vi "WildGruChil_V0.182.vi"() -> ()   [LabVIEW 2014]
uses:
  <vilib>/Utility/miscctls.llb/LVPointTypeDef.ctl
  <vilib>/Instr/_visa.llb/VISA Configure Serial Port (Instr).vi
  <vilib>/Utility/xml.llb/Read From XML File(string).vi
  <vilib>/Analysis/3filter.llb/IIR Filter (DBL).vi
  <vilib>/Utility/NIReport.llb/Append Report Text (str wrap).vi
  <vilib>/Utility/xml.llb/Write to XML File(string).vi
  <vilib>/Utility/NIReport.llb/NI_report.lvclass
  <vilib>/Analysis/NI_AALBase.lvlib
  <vilib>/gmath/NI_Gmath.lvlib
  <vilib>/Analysis/NI_AALPro.lvlib
panel:
  in  "min. Bytes":u32=15
  out "COM-Fehlerrate":string
  in  "nmax [1/min]":dbl=11000.0
  in  "nmin [1/min]":dbl=3000.0
  in  "Konfiguration:":bool
  in  "Speichern":bool
  in  "Drucken":bool
  out "Pmax":string="0,0 PS"
  in  "n vom Gas [1/min]":dbl=5000.0
  out "Ergebnis":string="0,0 PS bei 0 1/min   |   0,0 Nm bei 0 1/min   |   vmax: 2147483647 km/h\nDIN 70020 k =1,000 (20 °C, 50 %, 1013 mbar)\n20.11.2016 20:05 "
  in  "Fahrzeugdaten":string="Hier die Fahrzeugdaten eingeben"
  in  "Polynom":u8=15
  in  "Differenzenquotient":u8=12
  out "XY-Graph":cluster{dbl[], dbl[]}[](graph)
  in  "Rollenträgheit [kgm²]":dbl=0.402
  in  "[s]":dbl=5.0
  out "Untersetzung\nermittelt":bool
  out "Untersetzung":dbl format="%#.2f"
  in  "Reifenumfang [m]":dbl=1.222
  in  "Getriebe [1:]":dbl=5.343
  in  "Übersetzung ermitteln aus":bool=TRUE
  in  "Luftdruck [mbar]":dbl=1013.0
  in  "Luftfeuchtigkeit [%]":dbl=50.0
  in  "Lufttemperatur [°C]":dbl=20.0
  in  "Start [F1]":bool
  in  "Gl. Mittelwert":u8=35
  out "Füllstand Lesepuffer":u64(slide) scale=1.0..167.0
  out "Hinterrad\n[km/h]":dbl(knob) scale=0.0..150.0
  out "Welle\n[1/min]":cluster{dbl, dbl}(knob) scale=0.0..12000.0
  in  "Zündung [Imp/U]":u8=1
  in  "Rollenumfang [m]":dbl=0.613
  in  "Rolle [Inkr/U]":u16=200
  out "Lesepuffer":string="\n"
  in  "Serielle Schnittstelle":refnum<visa-resource-name>="COM6"
  in  "stop":bool
  out "Untersetzung-Graph":dbl(graph)=2.6802446808510636 caption="Untersetzung"
  # "1. n konstant halten\n2. START\n3. n weiter halten\n4. bei GO: Vollgas\n5. vom Gas gehen"
  # "Go"
  # "Zündsignal"
  # "Untersetzung:"
  # "Zündung\nRolle"
  # "Getriebe & Reifen"
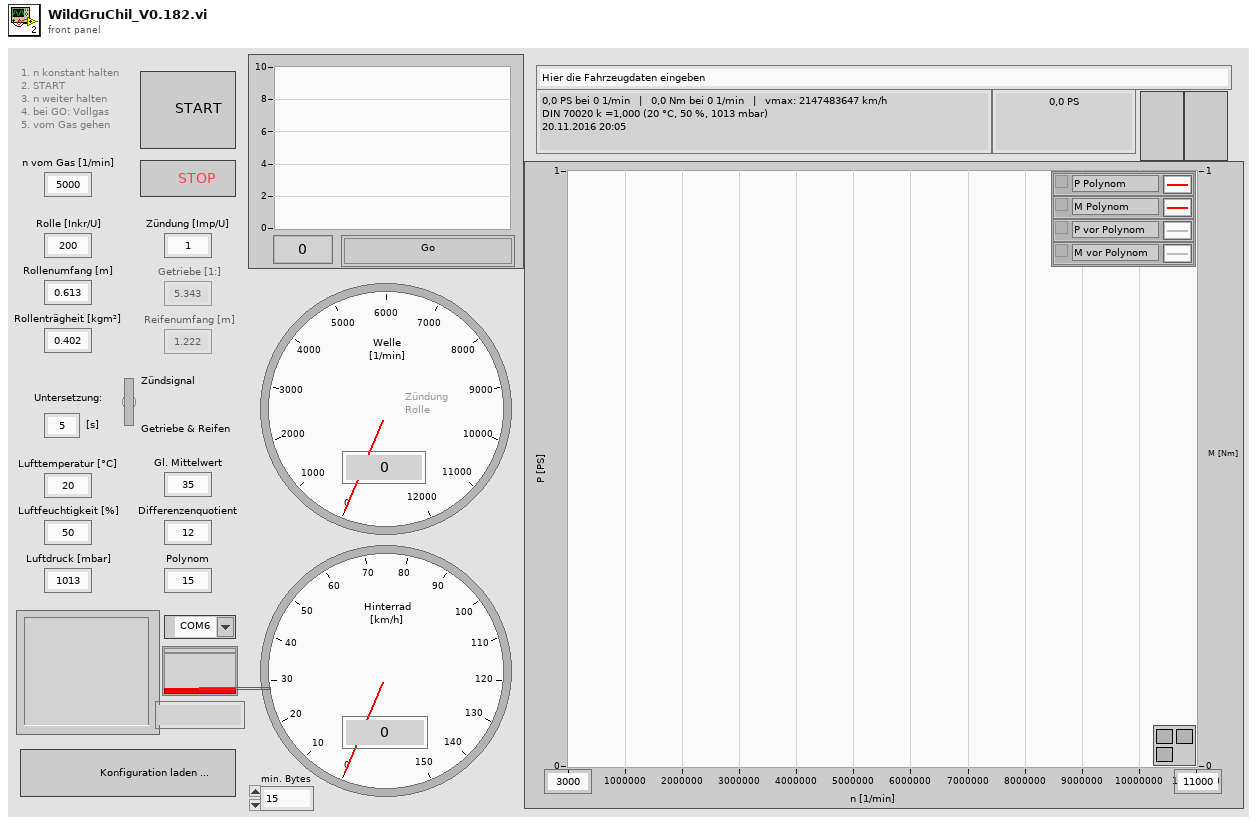
[diagram p1: front panel]
types:
  T1 = typedef "LVPointTypeDef.ctl" = cluster{"Horizontal":i16, "Vertical":i16}
  T2 = cluster{string, string, u16, dbl, dbl, u8, dbl, dbl, dbl, u8, u8, u8, dbl, dbl, dbl, dbl, dbl, dbl[], dbl[], dbl[], dbl[], bool, dbl, dbl, dbl, dbl, dbl[], i32[]}
  T3 = enum16{"Kleinste Quadrate", "Kleinestes absolutes Reiduum", "Biquadrat"}
  T4 = cluster{"Fahrzeugdaten":string, "date/time string":string, "Rolle [Inkr/U]":u16, "Rollenumfang [m]":dbl, "Rollenträgheit [kgm²]":dbl, "Zündung [Imp/U]":u8, "Getriebe [1:]":dbl, "Reifenumfang [m] ":dbl, "element":dbl, "Gl. Mittelwert":u8, "Differenzenquotient":u8, "Polynom":u8, "element":dbl, "element":dbl, "Lufttemperatur [°C]":dbl, "Luftfeuchtigkeit [%]":dbl, "Luftdruck [mbar]":dbl, dbl[], dbl[], "Best Polynomial Fit":dbl[], dbl[], "Übersetzung ermitteln aus":bool, "[s]":dbl, "nmin [1/min]":dbl, "nmax [1/min]":dbl, "n vom Gas [1/min]":dbl, dbl[], i32[]}
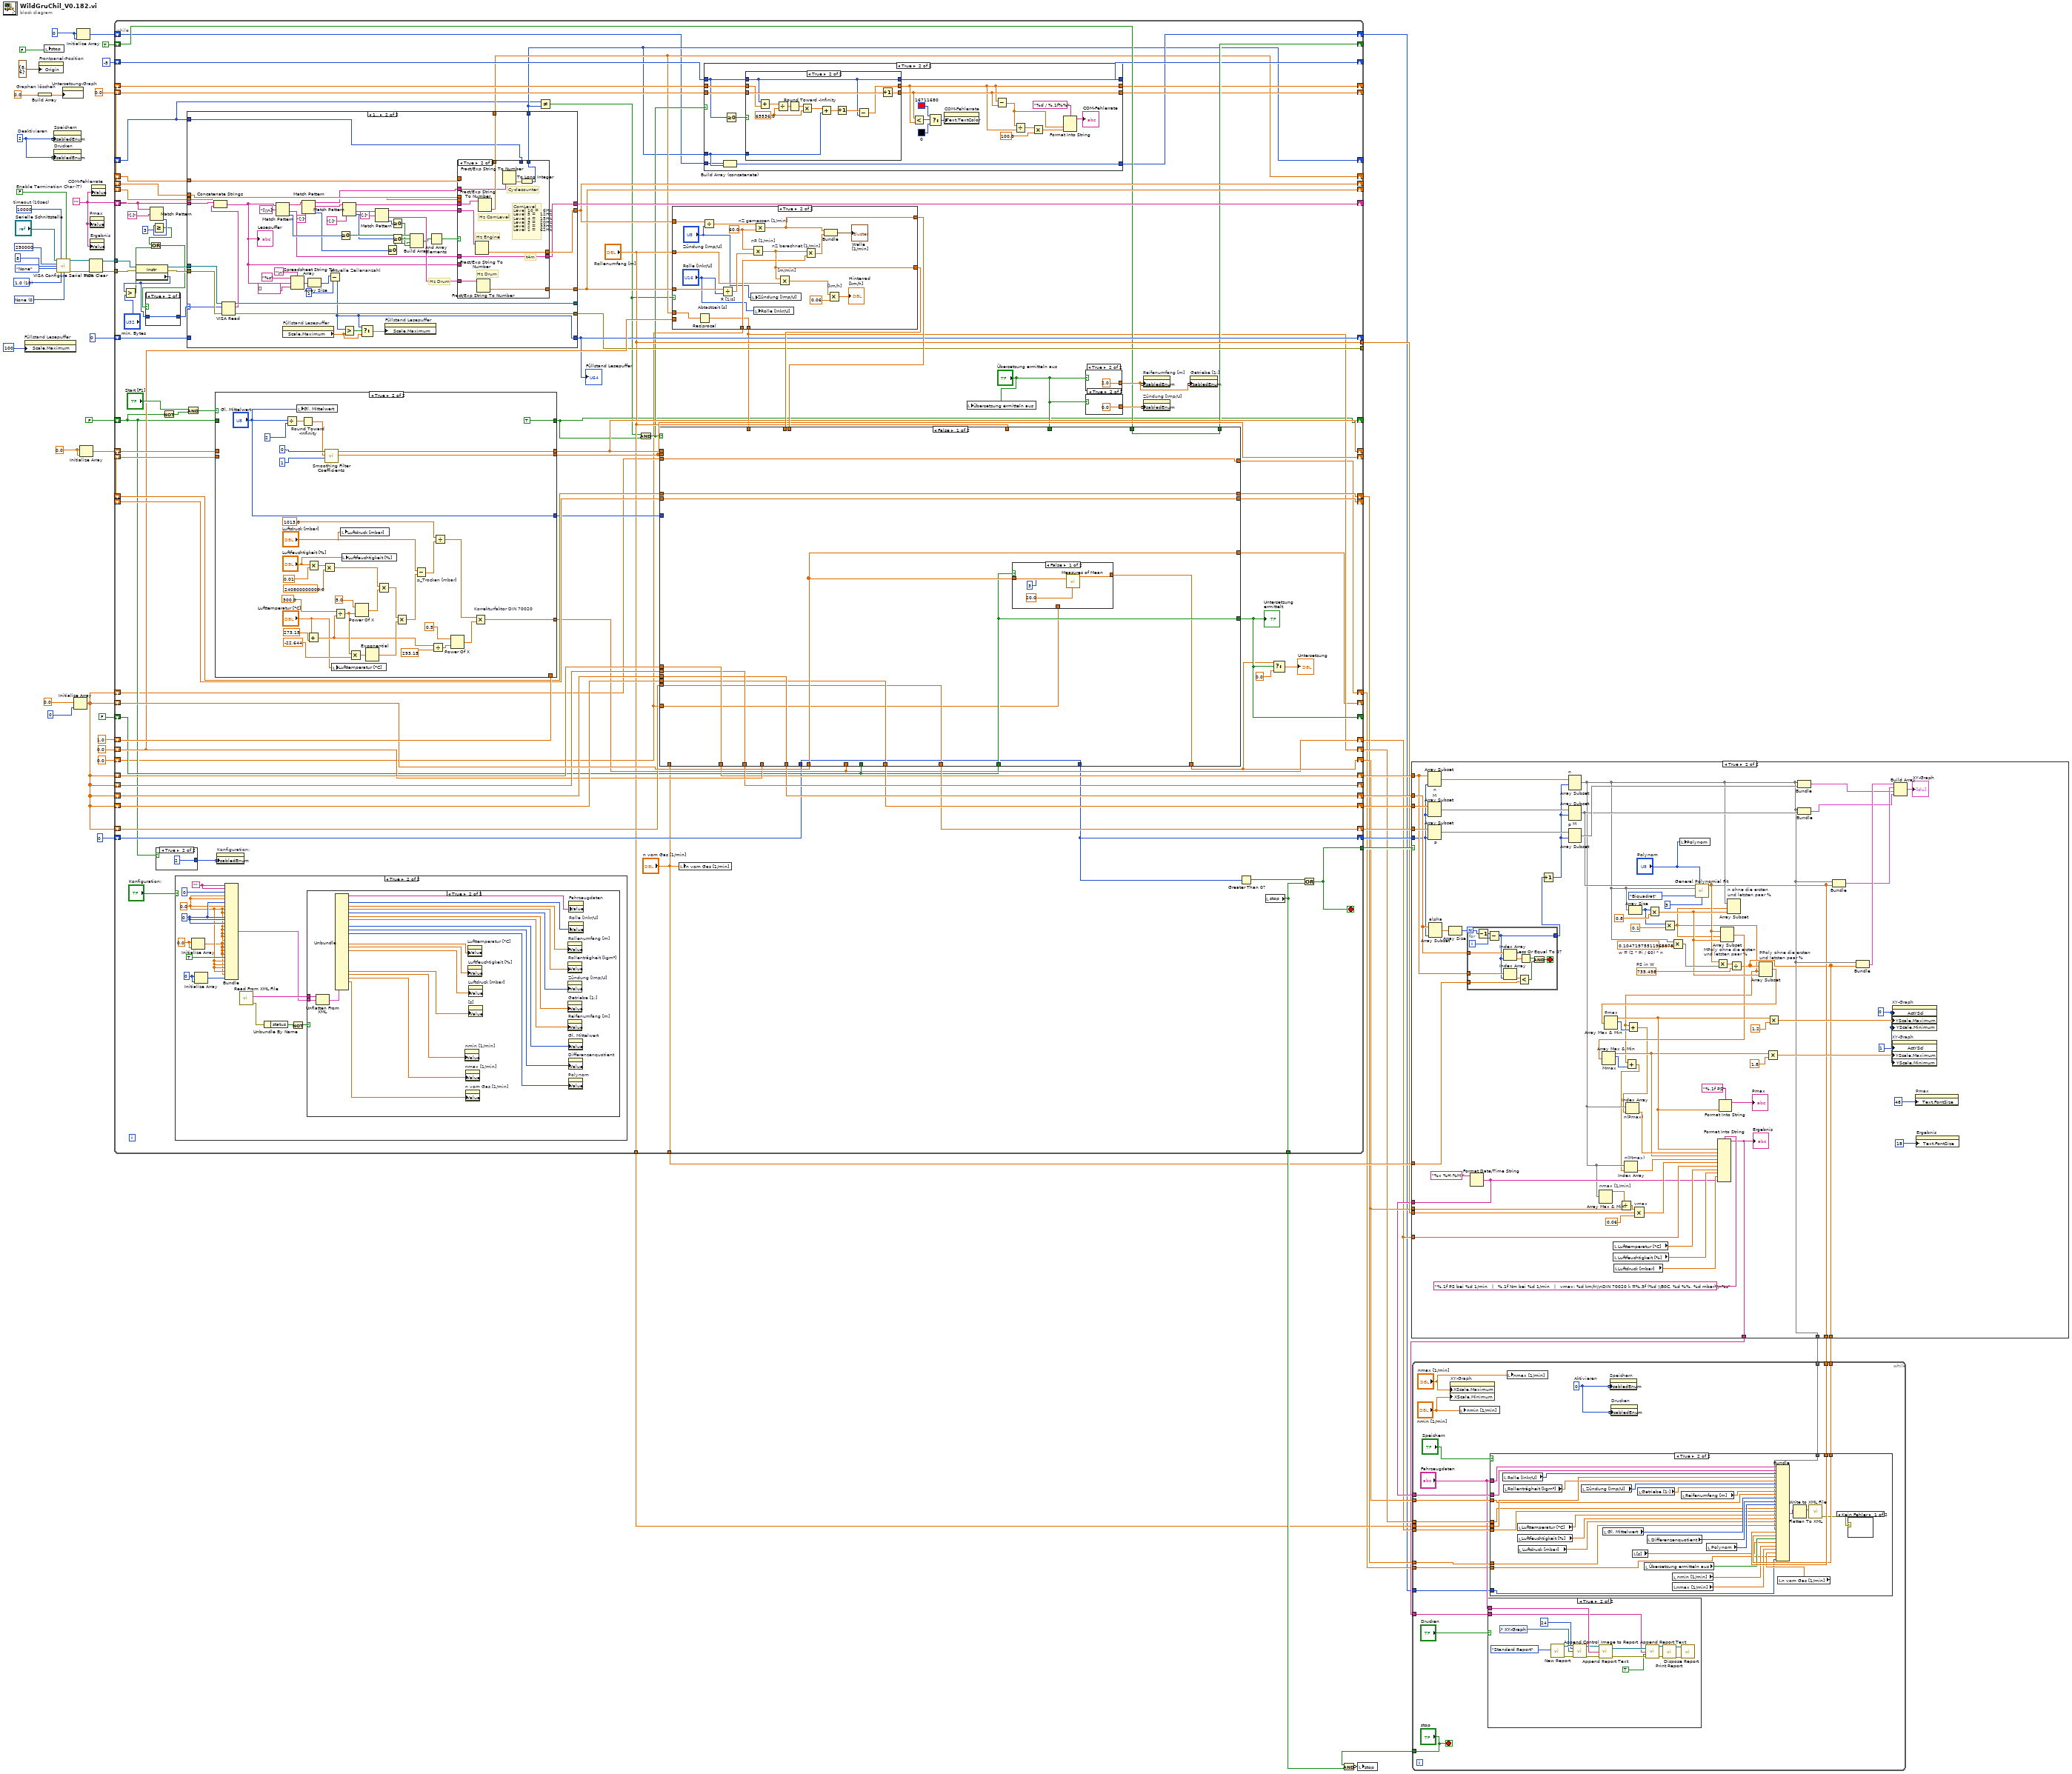
[diagram p0: block diagram]
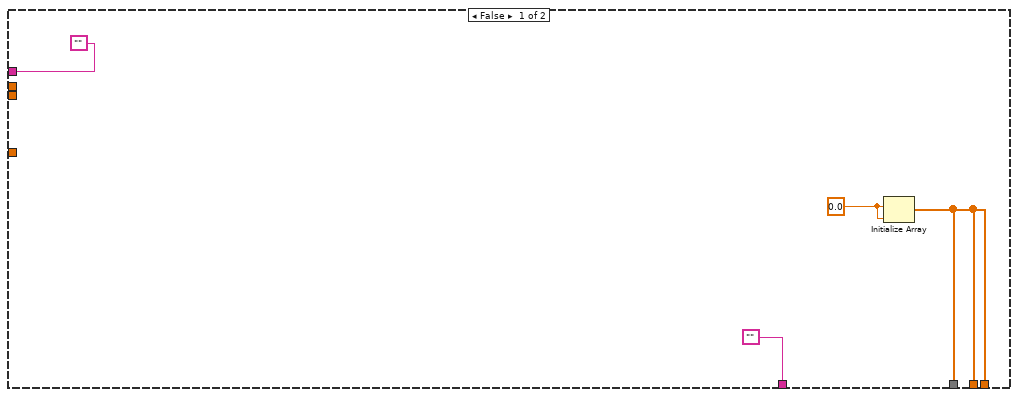
[diagram p5: hidden frame]
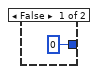
[diagram p6: hidden frame]
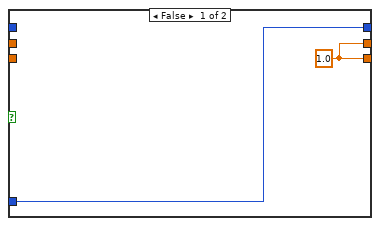
[diagram p8: hidden frame]
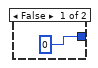
[diagram p11: hidden frame]
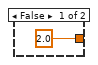
[diagram p12: hidden frame]
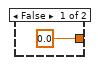
[diagram p13: hidden frame]
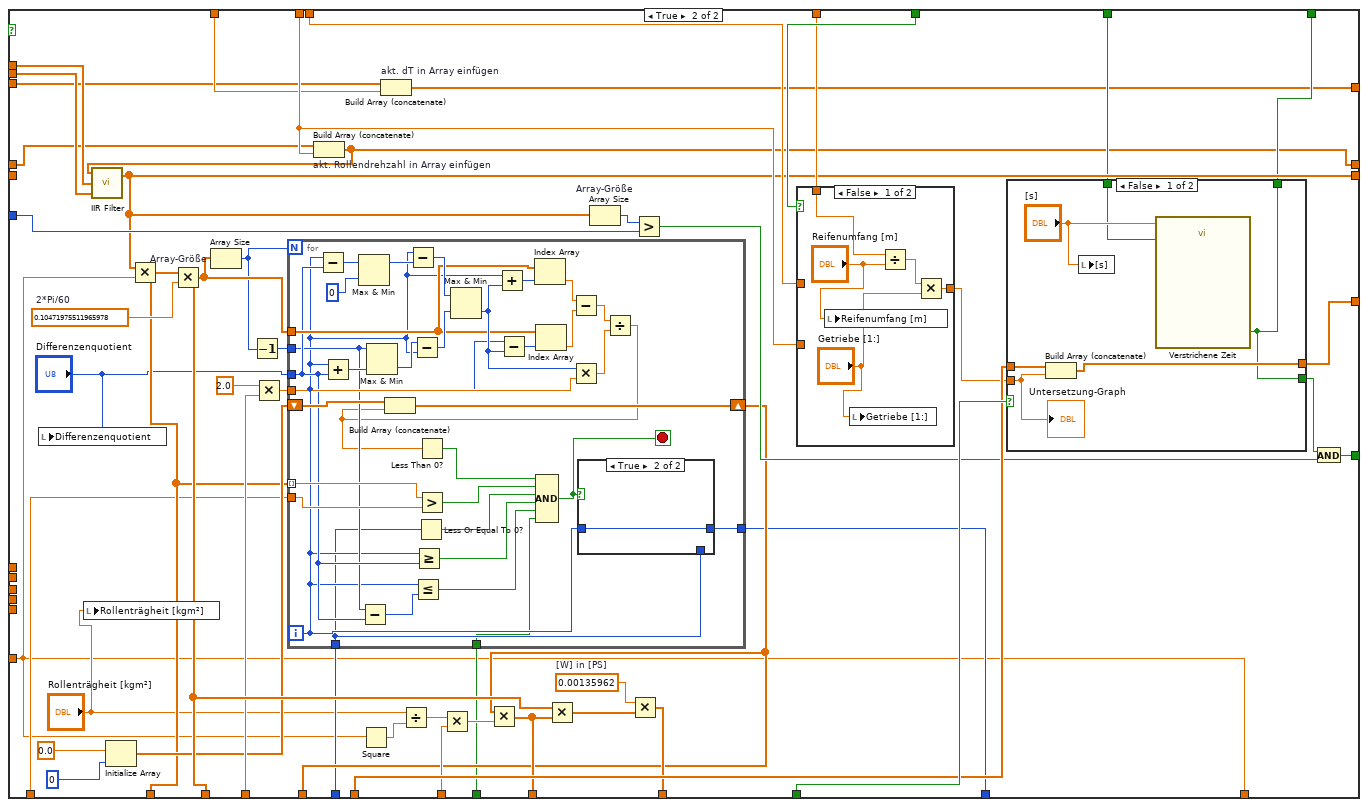
[diagram p15: hidden frame]
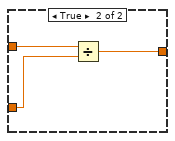
[diagram p18: hidden frame]
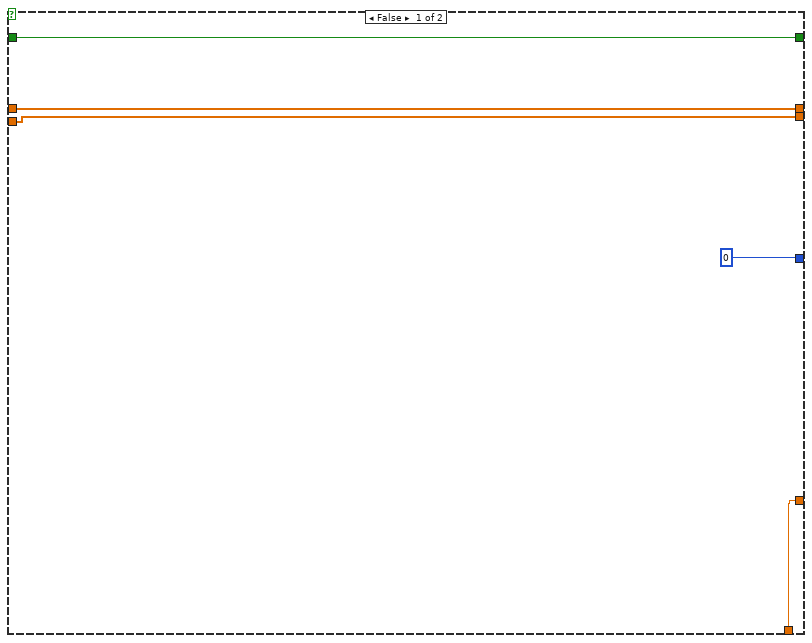
[diagram p19: hidden frame]
diagram:
  w6 = 0
  w2 = 0.0
  w11 = 2  # Deaktivieren
  w38 = 0.0
  w39 = 0.0  # Graphen löschen
  w54 = u16 0 items=["None", "XON/XOFF", "RTS/CTS", "XON/XOFF & RTS/CTS", "DTR/DSR", "XON/XOFF & DTR/DSR"] ("flow control (0:none)")
  w53 = u16 10 items=["1.0"=10, "1.5"=15, "2.0"=20] ("stop bits (10: 1 bit)")
  w3 = ""
  w58 = FALSE  # Enable Termination Char (T)
  w59 = u32 10000  # timeout (10sec)
  n1 = property on="Füllstand Lesepuffer" class="Schieber (strikt)"("Scale.Maximum"=100) -> ()  [unwired: 2 in, 2 out]
  n2 = Build Array(w39) -> (w36:dbl[])
  n3 = property on="Frontpanel-Position" class="Bereich"("Origin"=T1 {"Horizontal"=8, "Vertical"=6}) -> ()  [unwired: 2 in, 2 out]
  n4 = local write "stop"(FALSE) -> ()
  n5 = property on="Speichern" class="Bool."("DisabledEnum"=w11) -> ()  [unwired: 2 in, 2 out]
  n6 = property on="Drucken" class="Bool."("DisabledEnum"=w11) -> ()  [unwired: 2 in, 2 out]
  n7 = call-poly "VISA Configure Serial Port"("VISA resource name"="Serielle Schnittstelle", "timeout (10sec)"=w59, "Enable Termination\nChar (T)"=w58, "baud rate (9600)"=u32 250000 ("baudrate (250000)"), "data bits (8)"=u16 8, "parity (0:none)"=enum16{"None", "Odd", "Even", "Mark", "Space"}."None", "stop bits (10: 1 bit)"=w53, "flow control (0:none)"=w54) -> ("VISA resource name out"=w56:refnum<visa-resource-name>, "error out"=w57:errorcluster)  [unwired: 6 in]
  n8 = property on="Untersetzung-Graph" class="SVDiagr (strikt)"("History Data"=w36) -> ()  [unwired: 2 in, 2 out]
  n9 = Initialize Array(0.0 ("y"), 0) -> (w8:dbl[])
  n10 = Initialize Array(w6, w6) -> (w5:i32[])
  n11 = Initialize Array(w38, w38) -> (w37:dbl[])
  n12 = VISA Clear(VISA resource name=w56, error in (no error)=w57) -> (VISA resource name out=w51:refnum<visa-resource-name>, error out=w50:errorcluster)
  n13 = property on="Pmax" class="Str"("Value"=w3) -> ()  [unwired: 2 in, 2 out]
  n14 = property on="Ergebnis" class="Str"("Value"=w3) -> ()  [unwired: 2 in, 2 out]
  n15 = property on="COM-Fehlerrate" class="Str"("Value"=w3) -> ()  [unwired: 2 in, 2 out]
  n16 = while {
    tunnel: w51 -> [w149]
    tunnel: w50 -> [w148]
    shift-right: [w145] -> _
    shift-left: w3 -> [w65]
    shift-right: [w140] -> _
    shift-left: w2 -> [w144]
    shift-right: [w139] -> _
    shift-left: w2 -> [w143]
    shift-right: [w74] -> _
    shift-left: w2 -> [w142]
    shift-right: [w110] -> _
    shift-left: 0 -> [w141]
    shift-right: [w75] -> _
    shift-left: FALSE -> [w94]
    shift-right: [w105] -> w17
    shift-left: 1.0 ("element") -> [w133]
    shift-right: [w82] -> w22
    shift-left: 0.0 ("element") -> [w111]
    shift-right: [w126] -> w20
    shift-left: 0.0 ("element") -> [w77]
    shift-right: [w76] -> _
    shift-left: w8 -> [w130]
    shift-right: [w127] -> _
    shift-left: FALSE -> [w97]
    shift-right: [w125] -> _
    shift-left: w37 -> [w123]
    shift-right: [w124] -> _
    shift-left: w37 -> [w122]
    shift-right: [w121] -> w21
    shift-left: w37 -> [w119]
    shift-right: [w120] -> _
    shift-left: w37 -> [w118]
    shift-right: [w104] -> w29
    shift-left: w8 -> [w116]
    shift-right: [w109] -> _
    shift-left: w8 -> [w114]
    shift-right: [w108] -> w25
    shift-left: w8 -> [w115]
    shift-right: [w107] -> w28
    shift-left: w8 -> [w113]
    shift-right: [w106] -> w27
    shift-left: w8 -> [w112]
    tunnel: [w103] -> w35
    shift-right: [w98] -> w26
    shift-left: 0 -> [w100]
    tunnel: [w102] -> w31
    tunnel: [w101] -> _
    tunnel: ["n vom Gas [1/min]"] -> w24
    tunnel: ["Rollenumfang [m]"] -> w23
    tunnel: ["Rollenumfang [m]"] -> w15
    shift-right: [w89] -> _
    shift-left: TRUE -> [w90]
    shift-right: [w83] -> _
    shift-left: -5 -> [w88]
    shift-right: [w84] -> _
    shift-left: w2 -> [w87]
    shift-right: [w85] -> _
    shift-left: w2 -> [w86]
    shift-right: [w81] -> w7
    shift-left: w8 -> [w80]
    shift-right: [w73] -> _
    shift-left: _ -> [w72]
    shift-right: [w79] -> w4
    shift-left: w5 -> [w70]
    stop <- w103 stop-if-true
    n17 = property class="Instr"(reference=w149, error in=w148) -> (reference out=w146:refnum<visa-resource-name>, error out=w147:errorcluster, "Serial Settings:Number of Bytes at Serial Port"=w68:u32)
    n18 = Greater?(x=w68, y="min. Bytes") -> (0:w66:bool)
    n19 = Match Pattern(string=w65, regular expression="[;]") -> (offset past match=w63:i32)  [unwired: 1 in, 3 out]
    n20 = Greater Or Equal?(x=w63, y=3) -> (x >= y?=w62:bool)
    n21 = Or(x=w62, y=w66) -> (x .or. y?=w61:bool)
    n22 = case shown="True" w61 {
      tunnel: w68 -> [_ w151]
      tunnel: [u32 0 ("Bytes at Port") w151] -> w67
      frame False {
      }
      frame True {
      }
    }
    n23 = case shown="True" w94 {
      tunnel: [0 2] -> w93
      frame False {
      }
      frame True {
      }
    }
    n24 = Not(x=w94) -> (.not. x?=w138:bool)
    n25 = case shown="True" "Konfiguration:" {
      frame False {
      }
      frame True {
        w192 = 0
        w199 = u8 0
        w201 = 0.0
        w197 = 0.0
        w202 = ""
        n26 = Initialize Array(w201, w201) -> (w193:dbl[])
        n27 = Initialize Array(w192, w192) -> (w191:i32[])
        n28 = Bundle(w202, w202, u16 0, w197, w197, w199, w197, w197, w197, w199, w199, w199, w197, w197, w197, w197, w197, w193, w193, w193, w193, TRUE, w197, w197, w197, w197, w193, w191) -> (w203:T2)  [unwired: 1 in]
        n29 = call-poly <vilib>:"Read From XML File.vi"() -> ("error out"=w196:errorcluster, "XML Elements"=w204:string)  [unwired: 9 in, 1 out]
        n30 = Unbundle By Name(w196) -> ("status"=w194:bool)
        n31 = Not(x=w194) -> (.not. x?=w195:bool)
        n32 = case shown="True" w195 {
          tunnel: w204 -> [_ w224]
          tunnel: w203 -> [_ w223]
          frame False {
          }
          frame True {
            n33 = Unflatten From XML(xml string=w224, type=w223) -> (value=w222:T2)  [unwired: 1 in, 1 out]
            n34 = Unbundle(w222) -> (w221:string, w220:u16, w219:dbl, w218:dbl, w217:u8, w216:dbl, w215:dbl, w214:u8, w213:u8, w212:u8, w211:dbl, w210:dbl, w209:dbl, w208:dbl, w205:dbl, w206:dbl, w207:dbl)  [unwired: 11 out]
            n35 = property on="nmin [1/min]" class="DigWert (strikt)"("Value"=w205) -> ()  [unwired: 2 in, 2 out]
            n36 = property on="nmax [1/min]" class="DigWert (strikt)"("Value"=w206) -> ()  [unwired: 2 in, 2 out]
            n37 = property on="n vom Gas [1/min]" class="DigWert (strikt)"("Value"=w207) -> ()  [unwired: 2 in, 2 out]
            n38 = property on="Lufttemperatur [°C]" class="DigWert (strikt)"("Value"=w211) -> ()  [unwired: 2 in, 2 out]
            n39 = property on="Luftfeuchtigkeit [%]" class="DigWert (strikt)"("Value"=w210) -> ()  [unwired: 2 in, 2 out]
            n40 = property on="Luftdruck [mbar]" class="DigWert (strikt)"("Value"=w209) -> ()  [unwired: 2 in, 2 out]
            n41 = property on="[s]" class="DigWert (strikt)"("Value"=w208) -> ()  [unwired: 2 in, 2 out]
            n42 = property on="Rollenumfang [m]" class="DigWert (strikt)"("Value"=w219) -> ()  [unwired: 2 in, 2 out]
            n43 = property on="Rollenträgheit [kgm²]" class="DigWert (strikt)"("Value"=w218) -> ()  [unwired: 2 in, 2 out]
            n44 = property on="Zündung [Imp/U]" class="DigWert (strikt)"("Value"=w217) -> ()  [unwired: 2 in, 2 out]
            n45 = property on="Getriebe [1:]" class="DigWert (strikt)"("Value"=w216) -> ()  [unwired: 2 in, 2 out]
            n46 = property on="Reifenumfang [m]" class="DigWert (strikt)"("Value"=w215) -> ()  [unwired: 2 in, 2 out]
            n47 = property on="Gl. Mittelwert" class="DigWert (strikt)"("Value"=w214) -> ()  [unwired: 2 in, 2 out]
            n48 = property on="Differenzenquotient" class="DigWert (strikt)"("Value"=w213) -> ()  [unwired: 2 in, 2 out]
            n49 = property on="Polynom" class="DigWert (strikt)"("Value"=w212) -> ()  [unwired: 2 in, 2 out]
            n50 = property on="Fahrzeugdaten" class="Str"("Value"=w221) -> ()  [unwired: 2 in, 2 out]
            n51 = property on="Rolle [Inkr/U]" class="DigWert (strikt)"("Value"=w220) -> ()  [unwired: 2 in, 2 out]
          }
        }
      }
    }
    n52 = And(x="Start [F1]", y=w138) -> (x .and. y?=w137:bool)
    n53 = case shown="1.." w67 {
      selector: w67 -> [_ w463]
      tunnel: [w420 w457] -> w101
      tunnel: [w421 w458] -> _
      tunnel: w146 -> [w421 w465]
      tunnel: w147 -> [w420 w464]
      tunnel: [w417 w459] -> w139
      tunnel: [w418 w456] -> w140
      tunnel: w65 -> [w419 w454]
      tunnel: [w419 w452] -> w145
      tunnel: w144 -> [w418 w444]
      tunnel: w143 -> [w417 w443]
      tunnel: [w414 w442] -> w74
      tunnel: w142 -> [w414 w441]
      tunnel: w141 -> [w416 _]
      tunnel: [w416 w424] -> w110
      tunnel: [w415 w430] -> w73
      tunnel: w72 -> [w415 w429]
      frame 0, Default {
        # "No data in from serial port - Nothing to do."
      }
      frame 1.. {
        # "Hz Drum"
        n54 = VISA Read(VISA resource name=w465, byte count=w463, error in (no error)=w464) -> (VISA resource name out=w458:refnum<visa-resource-name>, read buffer=w455:string, error out=w457:errorcluster)  [unwired: 1 out]
        n55 = Concatenate Strings(w454, w455) -> (w426:string)
        "Lesepuffer" <- w426
        n56 = Match Pattern(string=w426, regular expression="[\\n]") -> (before substring=w433:string, after substring=w453:string, offset past match=w469:i32)  [unwired: 1 in, 1 out]
        n57 = property on="Füllstand Lesepuffer" class="Schieber (strikt)"() -> ("Scale.Maximum"=w423:dbl)  [unwired: 2 in, 2 out]
        n58 = Spreadsheet String To Array(delimiter (Tab)="\n" ("regular expression"), format string="%s" ("regular expression"), spreadsheet string=w426, array type (2D Dbl)=string[] [] ("Array 2")) -> (array=w435:string[])
        n59 = Match Pattern(string=w433, regular expression="[;]") -> (before substring=w431:string, after substring=w432:string, offset past match=w428:i32)  [unwired: 1 in, 1 out]
        n60 = Array Size(array=w435) -> (size(s)=w439:i32)
        n61 = Subtract "aktuelle Zeilenanzahl"(x=w439, y=1) -> (x-y=w424:i32)
        n62 = Greater Or Equal To 0?(x=w469) -> (x >= 0?=w451:bool)
        n63 = Match Pattern(string=w432, regular expression="[;]") -> (before substring=w462:string, after substring=w467:string, offset past match=w450:i32)  [unwired: 1 in, 1 out]
        n64 = Greater?(x=w424, y=w423) -> (0:w425:bool)
        n65 = Select(t=w424, s=w425, f=w423) -> (s? t:f=w422:dbl)
        n66 = Match Pattern(string=w467, regular expression="[;]") -> (before substring=w461:string, after substring=w460:string, offset past match=w448:i32)  [unwired: 1 in, 1 out]
        n67 = property on="Füllstand Lesepuffer" class="Schieber (strikt)"("Scale.Maximum"=w422) -> ()  [unwired: 2 in, 2 out]
        n68 = Greater Or Equal To 0?(x=w428) -> (x >= 0?=w427:bool)
        n69 = Greater Or Equal To 0?(x=w448) -> (x >= 0?=w447:bool)
        n70 = Greater Or Equal To 0?(x=w450) -> (x >= 0?=w449:bool)
        n71 = Build Array(w451, w449, w427, w447) -> (w446:bool[])
        n72 = And Array Elements(Boolean array=w446) -> (logical AND=w445:bool)
        n73 = case shown="True" w445 {
          tunnel: w462 -> [_ w480]
          tunnel: w461 -> [_ w485]
          tunnel: w460 -> [_ w484]
          tunnel: [w473 w483] -> w459
          tunnel: [w474 w482] -> w456
          tunnel: w453 -> [_ w481]
          tunnel: [w475 w481] -> w452
          tunnel: w426 -> [w475 _]
          tunnel: w444 -> [w474 _]
          tunnel: w443 -> [w473 _]
          tunnel: [w472 w479] -> w442
          tunnel: w441 -> [w472 _]
          tunnel: w431 -> [_ w478]
          tunnel: [w471 w476] -> w430
          tunnel: w429 -> [w471 _]
          frame False {
          }
          frame True {
            # "Cyclecounter"
            # "Hz ComLevel"
            # "ComLevel\nLevel 10 =   6Hz \nLevel 5 =   12Hz \nLevel 4 =   15Hz\nLevel 3 =   20Hz\nLevel 2 =   33Hz\nLevel 1 =   62Hz"
            # "Hz Drum"
            # "Hz Engine"
            # "t4m"
            n74 = Fract/Exp String To Number(string=w485) -> (number=w482:dbl)  [unwired: 3 in, 1 out]
            n75 = Fract/Exp String To Number(string=w484) -> (number=w483:dbl)  [unwired: 3 in, 1 out]
            n76 = Fract/Exp String To Number(string=w480) -> (number=w479:dbl)  [unwired: 3 in, 1 out]
            n77 = Fract/Exp String To Number(string=w478) -> (number=w477:dbl)  [unwired: 3 in, 1 out]
            n78 = To Long Integer(number=w477) -> (32bit integer=w476:i32)
          }
        }
      }
    }
    "Füllstand Lesepuffer" <- w110
    n79 = case shown="True" w137 {
      tunnel: [w357 TRUE] -> w75
      tunnel: w94 -> [w357 _]
      tunnel: [w356 w370] -> w105
      tunnel: w133 -> [w356 _]
      tunnel: [w355 w367] -> w125
      tunnel: [w354 w366] -> w124
      tunnel: w123 -> [w355 _]
      tunnel: w122 -> [w354 _]
      tunnel: [0 "Gl. Mittelwert"] -> w117
      frame False {
      }
      frame True {
        n80 = Divide(x="Gl. Mittelwert", y=2) -> (x/y=w365:dbl)
        n81 = local write "Gl. Mittelwert"("Gl. Mittelwert") -> ()
        n82 = Round Toward -Infinity(1:w365) -> (0:w364:dbl)
        n83 = Add(x="Lufttemperatur [°C]", y=273.15) -> (x+y=w376:dbl)
        n84 = Multiply(x="Luftfeuchtigkeit [%]", y=0.01) -> (x*y=w390:dbl)
        n85 = Multiply(x=w390, y=240800000000.0) -> (x*y=w361:dbl)
        n86 = call <vilib>:"Smoothing Filter Coefficients.vi"("shape"=1, "half-width"=w364, "type"=0) -> ("forward coefficients"=w366:dbl[], "reverse coefficients"=w367:dbl[])  [unwired: 6 in, 1 out]
        n87 = local write "Lufttemperatur [°C]"("Lufttemperatur [°C]") -> ()
        n88 = Divide ("M_Welle [Nm]")(x=300.0, y=w376) -> (x/y=w379:dbl)
        n89 = local write "Luftdruck [mbar]"("Luftdruck [mbar]") -> ()
        n90 = local write "Luftfeuchtigkeit [%]"("Luftfeuchtigkeit [%]") -> ()
        n91 = Multiply(x=w379, y=-22.644) -> (x*y=w385:dbl)
        n92 = Power Of X(1:w379, 2:5.0) -> (0:w377:dbl)
        n93 = Exponential(1:w385) -> (0:w383:dbl)
        n94 = Multiply(x=w361, y=w377) -> (x*y=w384:dbl)
        n95 = Multiply(x=w384, y=w383) -> (x*y=w382:dbl)
        n96 = Subtract "p_Trocken [mbar]"(x="Luftdruck [mbar]", y=w382) -> (x-y=w380:dbl)
        n97 = Divide ("M_Welle [Nm]")(x=w376, y=293.15) -> (x/y=w374:dbl)
        n98 = Divide ("M_Welle [Nm]")(x=1013.0, y=w380) -> (x/y=w372:dbl)
        n99 = Power Of X(1:w374, 2:0.5) -> (0:w371:dbl)
        n100 = Multiply "Korrekturfaktor DIN 70020"(x=w372, y=w371) -> (x*y=w370:dbl)
      }
    }
    n101 = property on="Konfiguration:" class="Bool."("DisabledEnum"=w93) -> ()  [unwired: 2 in, 2 out]
    n102 = Not Equal?(x=w72, y=w73) -> (x != y?=w71:bool)
    n103 = And(x=w71, y=w75) -> (x .and. y?=w78:bool)
    n104 = case "Case-Struktur" shown="True" w71 {
      tunnel: w140 -> [w395 w406]
      tunnel: w139 -> [w394 w405]
      tunnel: [w395 w404] -> w135
      tunnel: [w394 w403] -> w134
      tunnel: w74 -> [_ w397]
      tunnel: w111 -> [w393 _]
      tunnel: [w393 w396] -> w82
      tunnel: w77 -> [_ w402]
      tunnel: "Rollenumfang [m]" -> [_ w401]
      frame False {
      }
      frame True {
        w413 = 60.0 ("y")
        n105 = Reciprocal "Abtastzeit [s]"(x=w397) -> (1/x=w396:dbl)
        n106 = Divide(x=w406, y="Zündung [Imp/U]") -> (x/y=w409:dbl)
        n107 = Divide "R [1/s]"(x=w405, y="Rolle [Inkr/U]") -> (x/y=w412:dbl)
        n108 = local write "Zündung [Imp/U]"("Zündung [Imp/U]") -> ()
        n109 = Multiply "nR [1/min]"(x=w413, y=w412) -> (x*y=w403:dbl)
        n110 = Multiply "nZ gemessen [1/min]"(x=w409, y=w413) -> (x*y=w404:dbl)
        n111 = local write "Rolle [Inkr/U]"("Rolle [Inkr/U]") -> ()
        n112 = Multiply "[m/min]"(x=w403, y=w401) -> (x*y=w407:dbl)
        n113 = Multiply "nZ berechnet [1/min]"(x=w403, y=w402) -> (x*y=w411:dbl)
        n114 = Bundle(w404, w411) -> (→"Welle\n[1/min]":cluster{dbl, dbl})  [unwired: 1 in]
        n115 = Multiply "[km/h]"(x=w407, y=0.06) -> (x*y=→"Hinterrad\n[km/h]":dbl)
      }
    }
    n116 = case shown="False" w78 {
      tunnel: w135 -> [_ w291]
      tunnel: w134 -> [_ w290]
      tunnel: "Rollenumfang [m]" -> [_ w294]
      tunnel: [w242 w256] -> w126
      tunnel: w77 -> [w231 w256]
      tunnel: "Übersetzung ermitteln aus" -> [_ w299]
      tunnel: w97 -> [w243 w298]
      tunnel: w130 -> [w244 w297]
      tunnel: [w243 w268] -> w127
      tunnel: [w244 w296] -> w76
      tunnel: w125 -> [_ w293]
      tunnel: w124 -> [_ w292]
      tunnel: [w241 w253] -> w121
      tunnel: [w240 w267] -> w120
      tunnel: w119 -> [w241 w289]
      tunnel: w118 -> [w240 _]
      tunnel: w117 -> [_ w288]
      tunnel: [w239 w263] -> w104
      tunnel: w116 -> [w239 _]
      tunnel: [w238 w280] -> w109
      tunnel: w114 -> [w238 _]
      tunnel: w111 -> [_ w278]
      tunnel: [w237 w264] -> w108
      tunnel: w115 -> [w237 _]
      tunnel: [w236 w282] -> w107
      tunnel: w113 -> [w236 _]
      tunnel: [w235 w281] -> w106
      tunnel: w112 -> [w235 _]
      tunnel: w105 -> [_ w270]
      tunnel: w100 -> [w234 w262]
      tunnel: "n vom Gas [1/min]" -> [_ w261]
      tunnel: [w234 w260] -> w98
      tunnel: w97 -> [_ w259]
      tunnel: w90 -> [w233 w255]
      tunnel: [w233 w254] -> w89
      tunnel: w82 -> [_ w252]
      tunnel: [w232 w251] -> w81
      tunnel: w80 -> [w232 w250]
      frame False {
        n117 = case shown="False" w243 {
          tunnel: w244 -> [w248 _]
          tunnel: [w247 w249] -> w242
          tunnel: w231 -> [_ w249]
          frame False {
            n118 = call <vilib>:"Measures of Mean.vi"("percent (trim)"=20.0, "type"=3, "x array"=w248) -> ("mean value"=w247:dbl)  [unwired: 7 in, 1 out]
          }
          frame True {
          }
        }
      }
      frame True {
        w273 = 0.00135962  # [W] in [PS]
        w284 = 0.10471975511965978  # 2*Pi/60
        n119 = local write "Differenzenquotient"("Differenzenquotient") -> ()
        n120 = local write "Rollenträgheit [kgm²]"("Rollenträgheit [kgm²]") -> ()
        n121 = Initialize Array(0.0 ("y"), 0) -> (w274:dbl[])
        n122 = Multiply(x=2.0, y=w278) -> (x*y=w277:dbl)
        n123 = Build Array (concatenate) "akt. Rollendrehzahl in Array einfügen"(w289, w290) -> (w253:dbl[])
        n124 = call-poly <vilib>:"IIR Filter.vi"("Forward Coefficients"=w292, "Reverse Coefficients"=w293, "X"=w253) -> ("Filtered X"=w267:dbl[])  [unwired: 1 in, 1 out]
        n125 = Multiply(x=w267, y=w256) -> (x*y=w263:dbl[])
        n126 = Multiply(x=w263, y=w284) -> (x*y=w280:dbl[])
        n127 = Array Size "Array-Größe"(array=w280) -> (size(s)=w266:i32)
        n128 = Decrement(x=w266) -> (x-1=w265:i32)
        n129 = for {
          N: w266 -> [_]
          tunnel: "Differenzenquotient" -> [w311]
          tunnel: w280 -> [w319]
          tunnel: w265 -> [w310]
          tunnel: w277 -> [w320]
          shift-right: [w316] -> w264
          shift-left: w274 -> [w317]
          tunnel: w263 -> [w314] mode=indexing
          tunnel: w262 -> [w302]
          tunnel: w261 -> [w313]
          tunnel: [w303] -> w260
          tunnel: w259 -> [w300]
          i -> [w304]
          stop <- w301 stop-if-true
          n130 = Subtract(x=w304, y=w311) -> (x-y=w333:i32)
          n131 = Add(x=w304, y=w311) -> (x+y=w327:i32)
          n132 = Max & Min(x=w333, y=0) -> (max(x,y)=w331:i32)  [unwired: 1 out]
          n133 = Subtract(x=w310, y=w311) -> (x-y=w312:i32)
          n134 = Max & Min(x=w310, y=w327) -> (min(x,y)=w328:i32)  [unwired: 1 out]
          n135 = Subtract(x=w304, y=w331) -> (x-y=w330:i32)
          n136 = Subtract(x=w328, y=w304) -> (x-y=w329:i32)
          n137 = Less Or Equal?(x=w304, y=w312) -> (x <= y?=w308:bool)
          n138 = Greater Or Equal?(x=w304, y=w311) -> (x >= y?=w307:bool)
          n139 = Less Or Equal To 0?(x=w302) -> (x <= 0?=w305:bool)
          n140 = Greater?(x=w314, y=w313) -> (0:w315:bool)
          n141 = Max & Min(x=w330, y=w329) -> (min(x,y)=w321:i32)  [unwired: 1 out]
          n142 = Add(x=w304, y=w321) -> (x+y=w326:i32)
          n143 = Subtract(x=w304, y=w321) -> (x-y=w325:i32)
          n144 = Index Array(array=w319, index=w326) -> (element=w323:dbl)
          n145 = Index Array(array=w319, index=w325) -> (element=w324:dbl)
          n146 = Subtract(x=w323, y=w324) -> (x-y=w322:dbl)
          n147 = Multiply(x=w321, y=w320) -> (x*y=w318:dbl)
          n148 = Divide(x=w322, y=w318) -> (x/y=w309:dbl)
          n149 = Build Array (concatenate)(w317, w309) -> (w316:dbl[])
          n150 = Less Than 0?(x=w309) -> (x < 0?=w306:bool)
          n151 = Compound Arithmetic op=AND(w306, w315, w305, w307, w308, w300) -> (w301:bool)
          n152 = case shown="True" w301 {
            tunnel: w304 -> [_ w335]
            tunnel: [w334 w335] -> w303
            tunnel: w302 -> [w334 _]
            frame False {
            }
            frame True {
            }
          }
        }
        n153 = Square(x=w256) -> (x^2=w283:dbl)
        n154 = Build Array (concatenate) "akt. dT in Array einfügen"(w250, w252) -> (w251:dbl[])
        n155 = Divide(x="Rollenträgheit [kgm²]", y=w283) -> (x/y=w271:dbl)
        n156 = Multiply(x=w271, y=w270) -> (x*y=w269:dbl)
        n157 = Multiply(x=w264, y=w269) -> (x*y=w282:dbl[])
        n158 = Multiply(x=w280, y=w282) -> (x*y=w272:dbl[])
        n159 = Array Size "Array-Größe"(array=w267) -> (size(s)=w285:i32)
        n160 = Multiply(x=w273, y=w272) -> (x*y=w281:dbl[])
        n161 = Greater?(x=w285, y=w288) -> (0:w286:bool)
        n162 = case shown="False" w299 {
          tunnel: w291 -> [_ w352]
          tunnel: w290 -> [_ w351]
          tunnel: [w348 w350] -> w295
          tunnel: w294 -> [w349 _]
          frame False {
            n163 = local write "Reifenumfang [m]"("Reifenumfang [m]") -> ()
            n164 = local write "Getriebe [1:]"("Getriebe [1:]") -> ()
            n165 = Divide(x=w349, y="Reifenumfang [m]") -> (x/y=w347:dbl)
            n166 = Multiply(x=w347, y="Getriebe [1:]") -> (x*y=w348:dbl)
          }
          frame True {
            n167 = Divide(x=w352, y=w351) -> (x/y=w350:dbl)
          }
        }
        n168 = case shown="False" w298 {
          selector: w298 -> [_ w344]
          tunnel: w295 -> [w339 _]
          tunnel: w297 -> [w341 w343]
          tunnel: [w336 w344] -> w287
          tunnel: [w340 w343] -> w296
          tunnel: w255 -> [w337 w342]
          tunnel: [w336 w342] -> w254
          frame False {
            n169 = Build Array (concatenate)(w341, w339) -> (w340:dbl[])
            n170 = local write "[s]"("[s]") -> ()
            n171 = call "Verstrichene Zeit"("Time Target (s)"="[s]", "Reset"=w337) -> ("Time has Elapsed"=w336:bool)  [unwired: 10 in, 7 out]
            "Untersetzung-Graph" <- w339
          }
          frame True {
          }
        }
        n172 = And(x=w287, y=w286) -> (x .and. y?=w268:bool)
      }
    }
    "Untersetzung\nermittelt" <- w127
    n173 = local write "n vom Gas [1/min]"("n vom Gas [1/min]") -> ()
    n174 = case shown="True" w78 {
      tunnel: w88 -> [w155 w162]
      tunnel: [w155 w175] -> w83
      tunnel: w87 -> [w154 w174]
      tunnel: [w154 w158] -> w84
      tunnel: w86 -> [w153 w173]
      tunnel: [w153 w159] -> w85
      tunnel: w73 -> [_ w157]
      tunnel: w70 -> [w152 w156]
      tunnel: [w152 w161] -> w79
      frame False {
      }
      frame True {
        n175 = Build Array (concatenate)(w156, w157) -> (w161:i32[])
        n176 = Greater Or Equal To 0?(x=w162) -> (x >= 0?=w163:bool)
        n177 = case shown="True" w163 {
          tunnel: [w176 w187] -> w158
          tunnel: [w176 w188] -> w159
          tunnel: [w177 w179] -> w175
          tunnel: w174 -> [_ w181]
          tunnel: w173 -> [_ w189]
          tunnel: w157 -> [w177 w178]
          tunnel: w162 -> [_ w179]
          frame False {
            w176 = 1.0
          }
          frame True {
            w185 = 65536.0
            n178 = Add(x=w179, y=w181) -> (x+y=w180:dbl)
            n179 = Divide(x=w180, y=w185) -> (x/y=w190:dbl)
            n180 = Round Toward -Infinity(1:w190) -> (0:w186:dbl)
            n181 = Multiply(x=w186, y=w185) -> (x*y=w184:dbl)
            n182 = Add(x=w184, y=w178) -> (x+y=w183:dbl)
            n183 = Increment(x=w183) -> (x+1=w182:dbl)
            n184 = Subtract(x=w182, y=w179) -> (x-y=w187:dbl)
            n185 = Increment(x=w189) -> (x+1=w188:dbl)
          }
        }
        n186 = Less?(x=w159, y=w158) -> (x < y?=w171:bool)
        n187 = Select(t=u32 16711680, s=w171, f=u32 0) -> (s? t:f=w167:u32)
        n188 = property on="COM-Fehlerrate" class="Str"("Text.TextColor"=w167) -> ()  [unwired: 2 in, 2 out]
        n189 = Subtract(x=w158, y=w159) -> (x-y=w160:dbl)
        n190 = Divide(x=w160, y=w158) -> (x/y=w166:dbl)
        n191 = Multiply(x=w166, y=100.0) -> (x*y=w164:dbl)
        n192 = Format Into String(format string="%d / %.1f%%" ("Format-String"), w160, w164) -> (resulting string=→"COM-Fehlerrate":string)  [unwired: 2 in, 1 out]
      }
    }
    n193 = local write "Übersetzung ermitteln aus"("Übersetzung ermitteln aus") -> ()
    n194 = case shown="True" "Übersetzung ermitteln aus" {
      tunnel: [0.0 ("y") 2.0 ("y")] -> w131
      frame False {
      }
      frame True {
      }
    }
    n195 = case shown="True" "Übersetzung ermitteln aus" {
      tunnel: [2.0 ("y") 0.0 ("y")] -> w132
      frame False {
      }
      frame True {
      }
    }
    n196 = property on="Reifenumfang [m]" class="DigWert (strikt)"("DisabledEnum"=w131) -> ()  [unwired: 2 in, 2 out]
    n197 = property on="Zündung [Imp/U]" class="DigWert (strikt)"("DisabledEnum"=w132) -> ()  [unwired: 2 in, 2 out]
    n198 = property on="Getriebe [1:]" class="DigWert (strikt)"("DisabledEnum"=w131) -> ()  [unwired: 2 in, 2 out]
    n199 = Greater Than 0?(x=w98) -> (x > 0?=w99:bool)
    n200 = local read "stop"() -> (w102:bool)
    n201 = Select(t=w126, s=w127, f=0.0) -> (s? t:f=→"Untersetzung":dbl)
    n202 = Or(x=w99, y=w102) -> (x .or. y?=w103:bool)
  }
  n203 = case shown="True" w35 {
    tunnel: w29 -> [_ w547]
    tunnel: w28 -> [_ w552]
    tunnel: w27 -> [_ w551]
    tunnel: w26 -> [_ w523]
    tunnel: w25 -> [_ w548]
    tunnel: w24 -> [_ w546]
    tunnel: w23 -> [_ w540]
    tunnel: w17 -> [_ w526]
    tunnel: ["" w525] -> w18
    tunnel: w20 -> [_ w524]
    tunnel: ["" w522] -> w16
    tunnel: [w486 w499] -> w14
    tunnel: [w486 w498] -> w13
    tunnel: [w486 w497] -> w12
    frame False {
      w487 = 0.0
      n204 = Initialize Array(w487, w487) -> (w486:dbl[])
    }
    frame True {
      w511 = 735.498  # PS in W
      w517 = 0.10471975511965978  # w = (2 * Pi / 60) * n
      w521 = 0
      n205 = Array Subset "n"(array=w547, length=w523) -> (w545:dbl[])  [unwired: 1 in]
      n206 = Array Subset "M"(array=w552, length=w523) -> (w544:dbl[])  [unwired: 1 in]
      n207 = Array Subset "P"(array=w551, length=w523) -> (w543:dbl[])  [unwired: 1 in]
      n208 = Array Subset "alpha"(array=w548, length=w523) -> (w549:dbl[])  [unwired: 1 in]
      n209 = Array Size(array=w549) -> (size(s)=w550:i32)
      n210 = for {
        N: w550 -> [w570]
        tunnel: w548 -> [w567]
        tunnel: w547 -> [w564]
        tunnel: w546 -> [w561]
        tunnel: [w559] -> w519
        i -> [w565]
        stop <- w560 stop-if-true
        n211 = Decrement(x=w570) -> (x-1=w569:i32)
        n212 = Subtract(x=w569, y=w565) -> (x-y=w559:i32)
        n213 = Index Array(array=w567, index=w559) -> (element=w568:dbl)
        n214 = Index Array(array=w564, index=w559) -> (element=w563:dbl)
        n215 = Less?(x=w563, y=w561) -> (x < y?=w562:bool)
        n216 = Less Or Equal To 0?(x=w568) -> (x <= 0?=w566:bool)
        n217 = And(x=w566, y=w562) -> (x .and. y?=w560:bool)
      }
      n218 = Format Date/Time String(time format string (%c)="%x %H:%M ") -> (date/time string=w525:string)  [unwired: 2 in]
      n219 = Increment(x=w519) -> (x+1=w518:i32)
      n220 = Array Subset "n"(array=w545, index=w518) -> (w499:dbl[])  [unwired: 1 in]
      n221 = Array Subset "M"(array=w544, index=w518) -> (w516:dbl[])  [unwired: 1 in]
      n222 = Array Subset "P"(array=w543, index=w518) -> (w520:dbl[])  [unwired: 1 in]
      n223 = Array Max & Min "nmax [1/min]"(array=w499) -> (max value=w542:dbl)  [unwired: 3 out]
      n224 = local read "Lufttemperatur [°C]"() -> (w535:dbl)
      n225 = local read "Luftfeuchtigkeit [%]"() -> (w536:dbl)
      n226 = local read "Luftdruck [mbar]"() -> (w537:dbl)
      n227 = Divide(x=w542, y=w524) -> (x/y=w541:dbl)
      n228 = Array Size(array=w499) -> (size(s)=w496:i32)
      n229 = Compound Arithmetic op=MULTIPLY "vmax"(w541, w540, 0.06) -> (w532:dbl)
      n230 = Multiply(x=w496, y=0.8) -> (x*y=w507:dbl)
      n231 = Multiply(x=w496, y=0.1) -> (x*y=w490:dbl)
      n232 = Multiply(x=w499, y=w517) -> (x*y=w513:dbl[])
      n233 = local write "Polynom"("Polynom") -> ()
      n234 = call <vilib>:"General Polynomial Fit.vi"("Y"=w516, "polynomial order"="Polynom", "X"=w499, "method"=T3."Biquadrat" ("Methode"), "algorithm"=3) -> ("Best Polynomial Fit"=w498:dbl[])  [unwired: 7 in, 3 out]
      n235 = Multiply(x=w498, y=w513) -> (x*y=w512:dbl[])
      n236 = Array Subset "MPoly ohne die ersten\nund letzten paar %"(array=w498, index=w490, length=w507) -> (w501:dbl[])
      n237 = Array Max & Min "Mmax"(array=w501) -> (max value=w509:dbl, max index (indices)=w492:i32)  [unwired: 2 out]
      n238 = Add(x=w490, y=w492) -> (x+y=w491:dbl)
      n239 = Index Array "n(Mmax)"(array=w499, index=w491) -> (element=w533:dbl)
      n240 = Array Subset "n ohne die ersten \nund letzten paar %"(array=w499, index=w490, length=w507) -> ()  [unwired: 1 out]
      n241 = Divide(x=w512, y=w511) -> (x/y=w497:dbl[])
      n242 = Array Subset "PPoly ohne die ersten\nund letzten paar %"(array=w497, index=w490, length=w507) -> (w502:dbl[])
      n243 = Array Max & Min "Pmax"(array=w502) -> (max value=w510:dbl, max index (indices)=w494:i32)  [unwired: 2 out]
      n244 = Add(x=w490, y=w494) -> (x+y=w493:dbl)
      n245 = Index Array "n(Pmax)"(array=w499, index=w493) -> (element=w538:dbl)
      n246 = Format Into String(format string="%.1f PS bei %d 1/min   |   %.1f Nm bei %d 1/min   |   vmax: %d km/h\\nDIN 70020 k =%.3f (%d \\B0C, %d %%, %d mbar)\\n%s" ("Format-String"), w510, w538, w509, w533, w532, w526, w535, w536, w537, w525) -> (resulting string=w522:string)  [unwired: 2 in, 1 out]
      "Ergebnis" <- w522
      n247 = Format Into String(format string="%.1f PS" ("Format-String"), w510) -> (resulting string=→"Pmax":string)  [unwired: 2 in, 1 out]
      n248 = Multiply(x=w509, y=1.8) -> (x*y=w553:dbl)
      n249 = Multiply(x=w510, y=1.2) -> (x*y=w554:dbl)
      n250 = Bundle(w499, w520) -> (w503:cluster{dbl[], dbl[]})  [unwired: 1 in]
      n251 = Bundle(w499, w516) -> (w504:cluster{dbl[], dbl[]})  [unwired: 1 in]
      n252 = Bundle(w499, "Best Polynomial Fit"=w498) -> (w505:cluster{dbl[], "Best Polynomial Fit":dbl[]})  [unwired: 1 in]
      n253 = Bundle(w499, w497) -> (w506:cluster{dbl[], dbl[]})  [unwired: 1 in]
      n254 = property on="XY-Graph" class="XYGraph (strikt)"("ActYScl"=w521, "YScale.Maximum"=w554, "YScale.Minimum"=w521) -> ()  [unwired: 2 in, 2 out]
      n255 = property on="XY-Graph" class="XYGraph (strikt)"("ActYScl"=1, "YScale.Maximum"=w553, "YScale.Minimum"=w521) -> ()  [unwired: 2 in, 2 out]
      n256 = Build Array(w506, w505, w503, w504) -> (→"XY-Graph":cluster{dbl[], "Best Polynomial Fit":dbl[]}[])
      n257 = property on="Pmax" class="Str"("Text.FontSize"=48) -> ()  [unwired: 2 in, 2 out]
      n258 = property on="Ergebnis" class="Str"("Text.FontSize"=18) -> ()  [unwired: 2 in, 2 out]
    }
  }
  n259 = while {
    tunnel: ["stop"] -> w32
    tunnel: w20 -> [w587]
    tunnel: w22 -> [w586]
    tunnel: w17 -> [w585]
    tunnel: w21 -> [w584]
    tunnel: w18 -> [w583]
    tunnel: w16 -> [w580]
    tunnel: w15 -> [w579]
    tunnel: w14 -> [w578]
    tunnel: w13 -> [w577]
    tunnel: w12 -> [w576]
    tunnel: w7 -> [w572]
    tunnel: w4 -> [w571]
    stop <- "stop" stop-if-true
    w573 = 0  # Aktivieren
    n260 = property on="XY-Graph" class="XYGraph (strikt)"("XScale.Maximum"="nmax [1/min]", "XScale.Minimum"="nmin [1/min]") -> ()  [unwired: 2 in, 2 out]
    n261 = local write "nmin [1/min]"("nmin [1/min]") -> ()
    n262 = case shown="True" "Drucken" {
      tunnel: "Fahrzeugdaten" -> [_ w598]
      tunnel: w580 -> [_ w592]
      frame False {
      }
      frame True {
        n263 = control-ref of="XY-Graph"() -> (w600:refnum<vi>)
        n264 = call <vilib>:"New Report.vi"("report type"=enum16{"Standard Report", "HTML"}."Standard Report") -> ("report out"=w605:refnum<class "NI_report.lvclass">, "error out"=w604:errorcluster)  [unwired: 13 in]
        n265 = call-dynamic "Append Control Image to Report.vi"("report in"=w605, "image depth"=24, "ctrl reference"=w600, "error in (no error)"=w604) -> ("report out"=w597:refnum<class "NI_report.lvclass">, "error out"=w599:errorcluster)  [unwired: 8 in, 2 out]
        n266 = call-poly <vilib>:"Append Report Text.vi"("report in"=w597, "text"=w598, "error in (no error)"=w599) -> ("report out"=w596:refnum<class "NI_report.lvclass">, "error out"=w595:errorcluster)  [unwired: 9 in, 2 out]
        n267 = call-poly <vilib>:"Append Report Text.vi"("report in"=w596, "text"=w592, "append on new line? (F)"=TRUE, "error in (no error)"=w595) -> ("report out"=w594:refnum<class "NI_report.lvclass">, "error out"=w593:errorcluster)  [unwired: 8 in, 2 out]
        n268 = call-dynamic "Print Report.vi"("report in"=w594, "error in (no error)"=w593) -> ("report out"=w601:refnum<class "NI_report.lvclass">, "error out"=w602:errorcluster)  [unwired: 12 in]
        n269 = call-dynamic "Dispose Report.vi"("report in"=w601, "error in (no error)"=w602) -> ()  [unwired: 13 in, 1 out]
      }
    }
    n270 = case shown="True" "Speichern" {
      tunnel: w583 -> [_ w633]
      tunnel: w587 -> [_ w626]
      tunnel: w586 -> [_ w622]
      tunnel: w585 -> [_ w621]
      tunnel: w584 -> [_ w617]
      tunnel: "Fahrzeugdaten" -> [_ w634]
      tunnel: w579 -> [_ w631]
      tunnel: w578 -> [_ w616]
      tunnel: w577 -> [_ w615]
      tunnel: w576 -> [_ w614]
      tunnel: w572 -> [_ w607]
      tunnel: w571 -> [_ w606]
      frame False {
      }
      frame True {
        n271 = local read "Rolle [Inkr/U]"() -> (w632:u16)
        n272 = local read "Rollenträgheit [kgm²]"() -> (w630:dbl)
        n273 = local read "Lufttemperatur [°C]"() -> (w620:dbl)
        n274 = local read "Luftfeuchtigkeit [%]"() -> (w619:dbl)
        n275 = local read "Luftdruck [mbar]"() -> (w618:dbl)
        n276 = local read "Zündung [Imp/U]"() -> (w629:u8)
        n277 = local read "Gl. Mittelwert"() -> (w625:u8)
        n278 = local read "[s]"() -> (w612:dbl)
        n279 = local read "Getriebe [1:]"() -> (w628:dbl)
        n280 = local read "Übersetzung ermitteln aus"() -> (w613:bool)
        n281 = local read "Differenzenquotient"() -> (w624:u8)
        n282 = local read "nmax [1/min]"() -> (w610:dbl)
        n283 = local read "nmin [1/min]"() -> (w611:dbl)
        n284 = local read "Reifenumfang [m]"() -> (w627:dbl)
        n285 = local read "Polynom"() -> (w623:u8)
        n286 = local read "n vom Gas [1/min]"() -> (w609:dbl)
        n287 = Bundle("Fahrzeugdaten"=w634, "date/time string"=w633, "Rolle [Inkr/U]"=w632, "Rollenumfang [m]"=w631, "Rollenträgheit [kgm²]"=w630, "Zündung [Imp/U]"=w629, "Getriebe [1:]"=w628, "Reifenumfang [m]"=w627, "element"=w626, "Gl. Mittelwert"=w625, "Differenzenquotient"=w624, "Polynom"=w623, "element"=w622, "element"=w621, "Lufttemperatur [°C]"=w620, "Luftfeuchtigkeit [%]"=w619, "Luftdruck [mbar]"=w618, w617, w616, "Best Polynomial Fit"=w615, w614, "Übersetzung ermitteln aus"=w613, "[s]"=w612, "nmin [1/min]"=w611, "nmax [1/min]"=w610, "n vom Gas [1/min]"=w609, w607, w606) -> (w636:T4)  [unwired: 1 in]
        n288 = Flatten To XML(anything=w636) -> (xml string=w635:string)
        n289 = call-poly <vilib>:"Write to XML File.vi"("XML Input"=w635) -> ("error out"=w608:errorcluster)  [unwired: 8 in, 2 out]
        n290 = case shown="Kein Fehler" w608 {
          frame No Error {
          }
          frame Error {
          }
        }
      }
    }
    n291 = local write "nmax [1/min]"("nmax [1/min]") -> ()
    n292 = property on="Speichern" class="Bool."("DisabledEnum"=w573) -> ()  [unwired: 2 in, 2 out]
    n293 = property on="Drucken" class="Bool."("DisabledEnum"=w573) -> ()  [unwired: 2 in, 2 out]
  }
  n294 = Compound Arithmetic op=AND(w32, w31) -> (invert w19:bool)
  n295 = local write "stop"(w19) -> ()
